vi "Recurse.vi"(0 "Combo index in":i32, 1 "Iterations array in":i32[](array[numeric]), 2 "Quantities":i32[](array[numeric]), 3 "Update display?":bool, 5 "Combos in":i32[][](array[numeric]), 7 "Values":i32[](array[numeric]), 9 "Goal amount":i32, 11 "Depth":i32, 12 "Result index in":i32, 13 "Results in":i32[][](array[numeric])) -> (4 "Progress - current iteration values":i32[](array[numeric]), 6 "Combo index out":i32, 8 "Combos out":i32[][](array[numeric]), 10 "Result index out":i32, 14 "Results out":i32[][](array[numeric]))   [LabVIEW 2014]
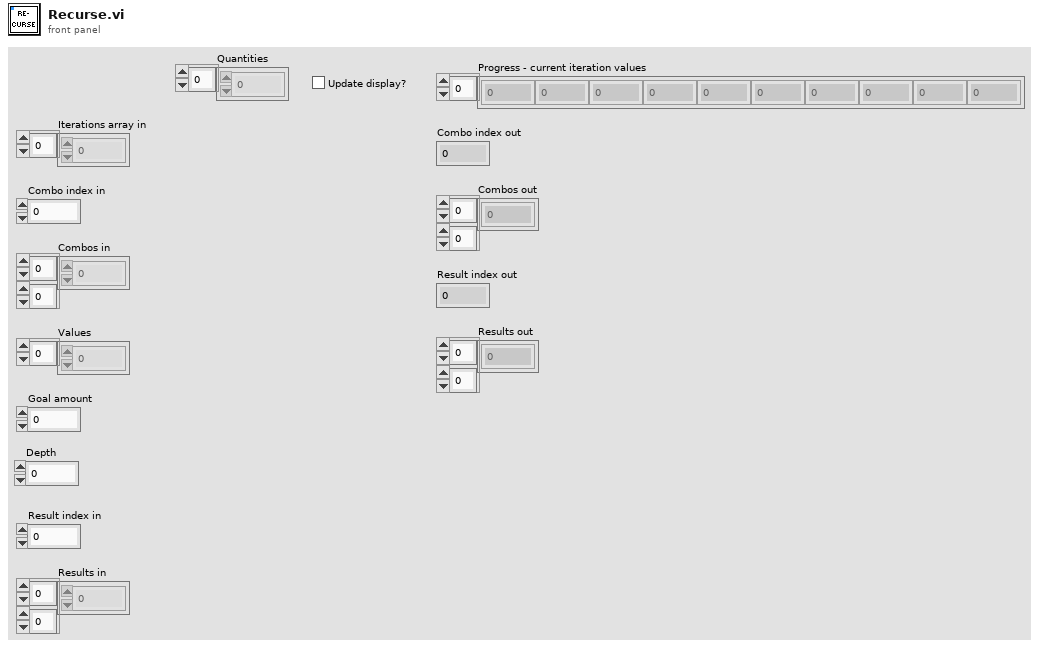
[diagram p1: front panel]
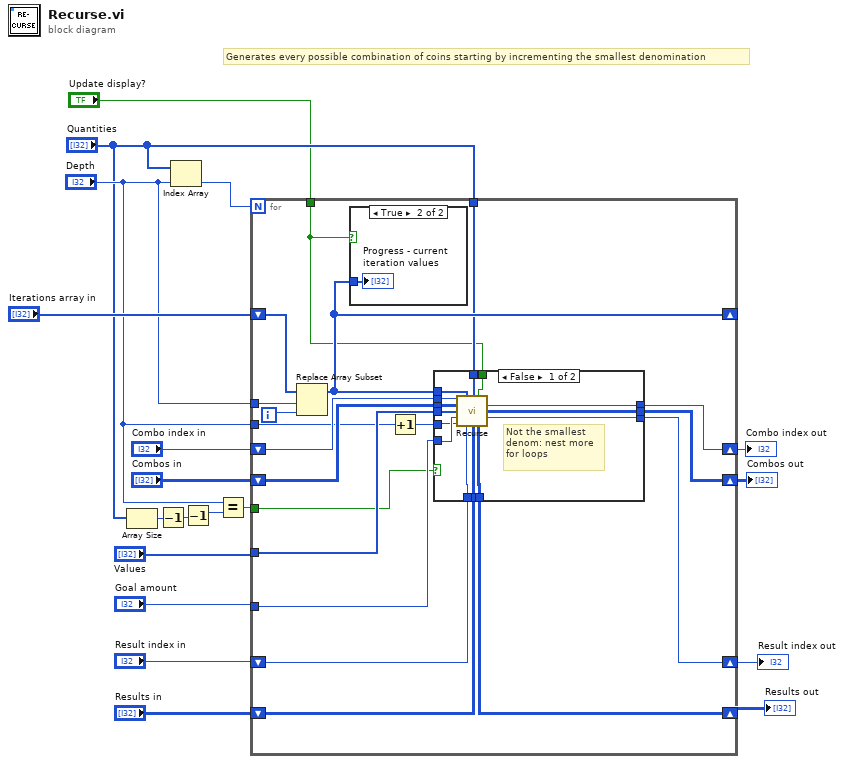
[diagram p0: block diagram]
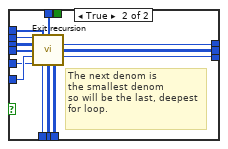
[diagram p3: hidden frame]
diagram:
  # "Generates every possible combination of coins starting by incrementing the smallest denomination"
  n1 = Array Size(array="Quantities") -> (size(s)=w4:i32)
  n2 = Decrement(x=w4) -> (x-1=w3:i32)
  n3 = Index Array(array="Quantities", index="Depth") -> (element=w8:i32)
  n4 = Decrement(x=w3) -> (x-1=w2:i32)
  n5 = Equal?(x="Depth", y=w2) -> (x = y?=w5:bool)
  n6 = for {
    N: w8 -> [_]
    shift-right: [w24] -> w9
    shift-left: "Combos in" -> [w38]
    shift-right: [w25] -> w12
    shift-left: "Combo index in" -> [w37]
    tunnel: "Values" -> [w30]
    shift-right: [w26] -> w17
    shift-left: "Result index in" -> [w27]
    shift-right: [w28] -> w16
    shift-left: "Results in" -> [w36]
    shift-right: [w32] -> _
    shift-left: "Iterations array in" -> [w33]
    tunnel: "Goal amount" -> [w29]
    tunnel: "Depth" -> [w34]
    tunnel: "Quantities" -> [w31]
    tunnel: "Depth" -> [w22]
    tunnel: w5 -> [w21]
    tunnel: "Update display?" -> [w20]
    i -> [w35]
    n7 = Replace Array Subset(array=w33, new element=w35, index=w34) -> (w32:i32[])
    n8 = case shown="True" w20 {
      tunnel: w32 -> [_ w39]
      frame False {
      }
      frame True {
        "Progress - current iteration values" <- w39
      }
    }
    n9 = Increment(x=w22) -> (x+1=w23:i32)
    n10 = case shown="False" w21 {
      tunnel: w38 -> [w50 w66]
      tunnel: w37 -> [w51 w65]
      tunnel: w36 -> [w48 w64]
      tunnel: w32 -> [w52 w63]
      tunnel: w31 -> [w53 w62]
      tunnel: w30 -> [w45 w61]
      tunnel: w29 -> [w44 w60]
      tunnel: [w47 w59] -> w28
      tunnel: w27 -> [w49 w58]
      tunnel: [w46 w57] -> w26
      tunnel: [w42 w56] -> w25
      tunnel: [w41 w55] -> w24
      tunnel: w23 -> [w43 w54]
      tunnel: w20 -> [w40 _]
      frame False {
        # "Not the smallest\ndenom: nest more\nfor loops"
        n11 = call "Recurse.vi"("Combo index in"=w51, "Iterations array in"=w52, "Quantities"=w53, "Update display?"=w40, "Combos in"=w50, "Values"=w45, "Goal amount"=w44, "Depth"=w43, "Result index in"=w49, "Results in"=w48) -> ("Combo index out"=w42:i32, "Combos out"=w41:i32[][], "Result index out"=w46:i32, "Results out"=w47:i32[][])  [unwired: 1 in, 1 out]
      }
      frame True {
        # "The next denom is\nthe smallest denom\nso will be the last, deepest\nfor loop."
        n12 = call "Exit recursion.vi"("combo index in"=w65, "Iterations array in"=w63, "Quantities"=w62, "Combos in"=w66, "Values"=w61, "Goal amount"=w60, "Depth"=w54, "Result index in"=w58, "Results in"=w64) -> ("Combo index out"=w56:i32, "Combos out"=w55:i32[][], "Result index out"=w57:i32, "Results out"=w59:i32[][])  [unwired: 2 in, 1 out]
      }
    }
  }
  "Result index out" <- w17
  "Results out" <- w16
  "Combo index out" <- w12
  "Combos out" <- w9
